vi "FieldDisp_Read_Field_Pic.vi"(11 "file name":string) -> (0 "Image Error":errorcluster, 1 "Image Out":T1, 2 "Picture Error":errorcluster, 3 "Picture Data":T2)   [LabVIEW 2019, in "Trajectory_Library.lvlib"]
doc: "Internal function -- should not be called directly by users.\n\nCompelte documentation TBD."
uses:
  Trajectory_Library.lvlib
  <vilib>/picture/picture.llb/imagedata.ctl
  <vilib>/vision/Image Controls.llb/IMAQ Image.ctl
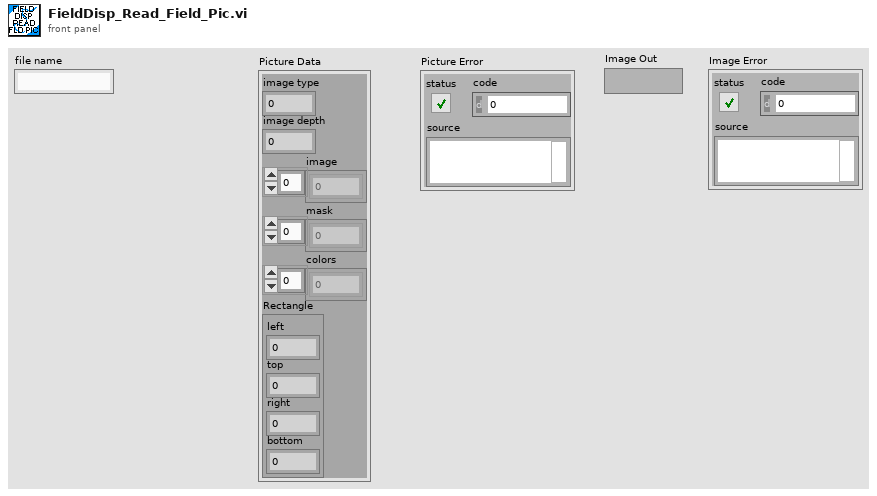
[diagram p1: front panel]
types:
  T1 = typedef "IMAQ Image.ctl" = refnum<image>
  T2 = typedef "imagedata.ctl" = cluster{"image type":i32, "image depth":i32, "image":u8[], "mask":u8[], "colors":u32[], "Rectangle":cluster{"left":i16, "top":i16, "right":i16, "bottom":i16}}
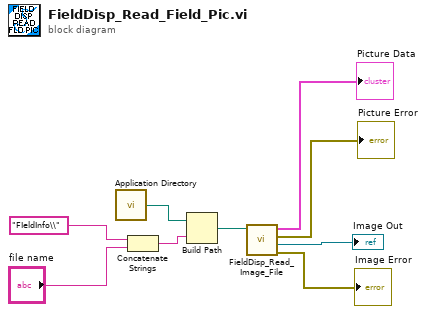
[diagram p0: block diagram]
diagram:
  n1 = call <vilib>:"Application Directory.vi"() -> ("Application Directory"=w5:path)
  n2 = Concatenate Strings("FIeldInfo\\" ("string"), "file name") -> (w9:string)
  n3 = Build Path(base path=w5, name or relative path=w9) -> (appended path=w6:path)
  n4 = call "FieldDisp_Read_Image_File.vi"("file"=w6) -> ("Image Error"=→"Image Error":errorcluster, "Image Out"=→"Image Out":T1, "Picture Error"=→"Picture Error":errorcluster, "Picture Data"=→"Picture Data":T2)  [unwired: 7 in]
